vi "Property Strings.vi"() -> ()   [LabVIEW 2016, in "Scan Engine Custom Device.lvlib"]
uses:
  Scan Engine Custom Device.lvlib
panel:
  in  "Host IP":string="FPGALoadDelay"
  in  "SW Index":string="SW Index"
  in  "CW Index":string="CW Index"
  in  "DS402-Status":string="DS402-Status"
  in  "DS402-Commands":string="DS402-Commands"
  in  "Status Variables":string="Status Variables"
  in  "Outputs of ECAT Slave":string="Outputs of ECAT Slave"
  in  "Inputs for ECAT Slave":string="Inputs for ECAT Slave"
  in  "I/O Network Variables":string="I/O Network Variables"
  in  "FPGALoadDelay":string="FPGALoadDelay"
  in  "ECAT Slave Prepend":string="ECAT Slave Prepend"
  in  "IOVarName":string="IOVarName"
  in  "# Slots":string="# Slots"
  in  "Async Decimation":string="Async Decimation"
  in  "Cyclic Data Bandwidth":string="Cyclic Data Bandwidth"
  in  "Bitfile Path - Target":string="Bitfile Path - Target"
  in  "Bitfile Path - Host":string="Bitfile Path - Host"
  in  "FPGA Target":string="FPGA Target"
  in  "FPGA Sig":string="FPGA Sig"
  in  "FXP Config":string="FXP Config"
  in  "Data Type":string="Data Type"
  in  "Product Code":string="Product Code"
  in  "ECAT Master ID":string="ECAT Master ID"
  in  "ECAT Slave #":string="ECAT Slave #"
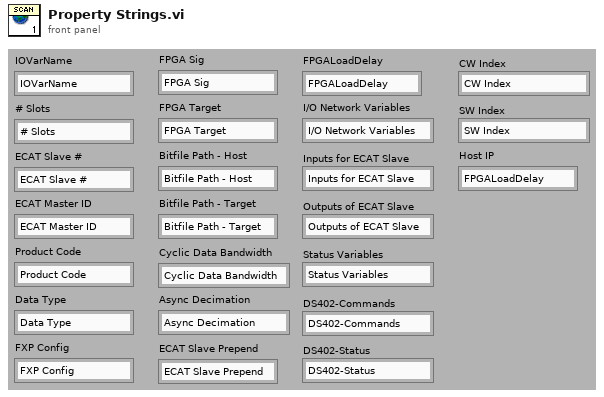
[diagram p1: front panel]
diagram:
